vi "Lift Catch.vi"(9 "encLiftRate":dbl, 11 "inLoop":bool) -> ()   [LabVIEW 2014]
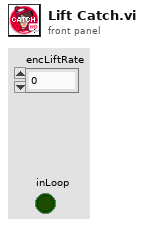
[diagram p1: front panel]
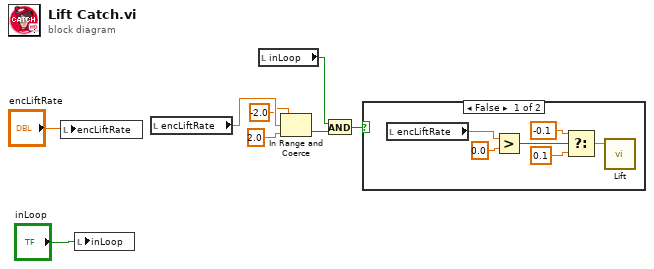
[diagram p0: block diagram]
diagram:
  n1 = local write "encLiftRate"("encLiftRate") -> ()
  n2 = local write "inLoop"("inLoop") -> ()
  n3 = local read "encLiftRate"() -> (w3:dbl)
  n4 = local read "inLoop"() -> (w2:bool)
  n5 = In Range and Coerce(upper limit=-2.0, x=w3, lower limit=2.0) -> (In Range?=w6:bool)  [unwired: 1 out]
  n6 = And(x=w2, y=w6) -> (x .and. y?=w8:bool)
  n7 = case shown="False" w8 {
    frame False {
      n8 = local read "encLiftRate"() -> (w9:dbl)
      n9 = Greater?(x=w9, y=0.0) -> (0:w13:bool)
      n10 = Select(t=-0.1, s=w13, f=0.1) -> (s? t:f=w14:dbl)
      n11 = call "Lift.vi"("Power Value"=w14) -> ()  [unwired: 11 in]
    }
    frame True {
    }
  }
